vi "2B_Tech_TCP_Packet_TWBOZO_v1.1.vi"(7 "TCP Packet In":string, 12 "Data Array":string[](array[string])) -> (8 "TCP Binary Packet":string)   [LabVIEW 2014]
panel:
  out "array":string[](array[string])
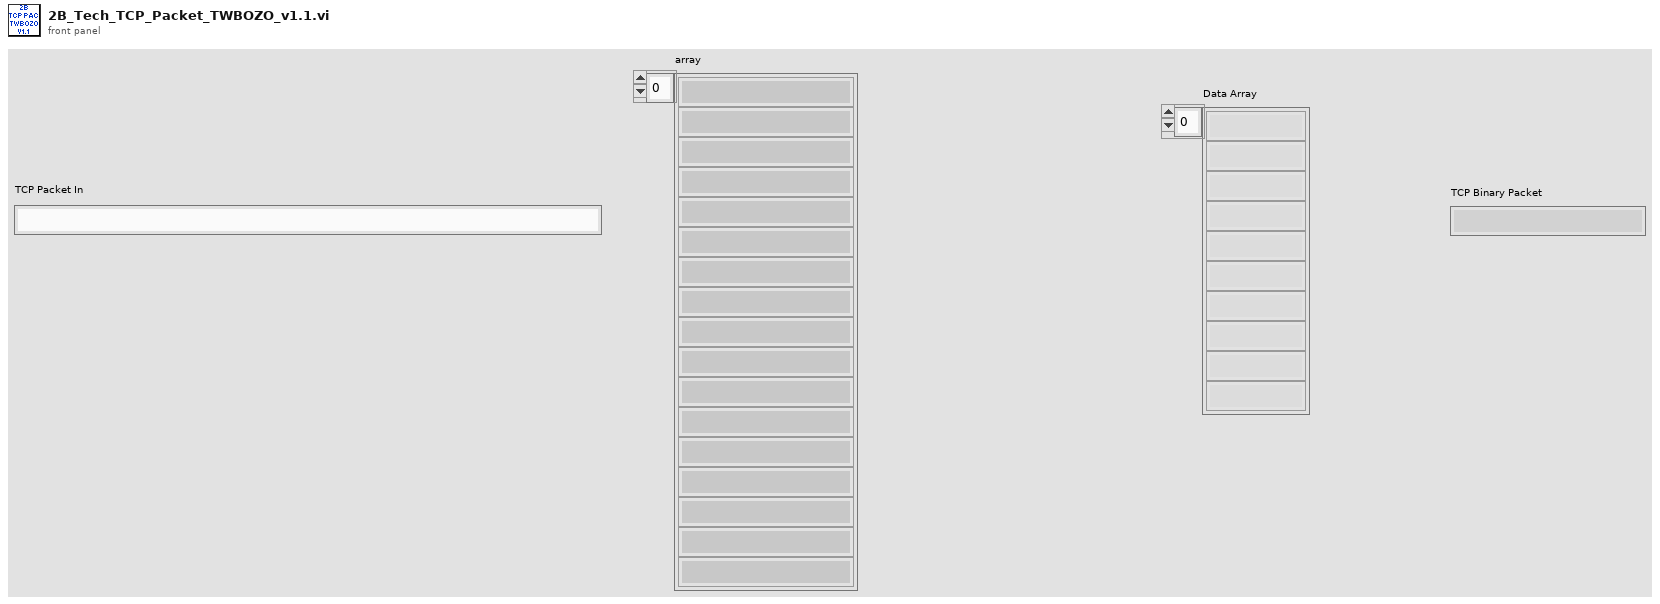
[diagram p1: front panel]
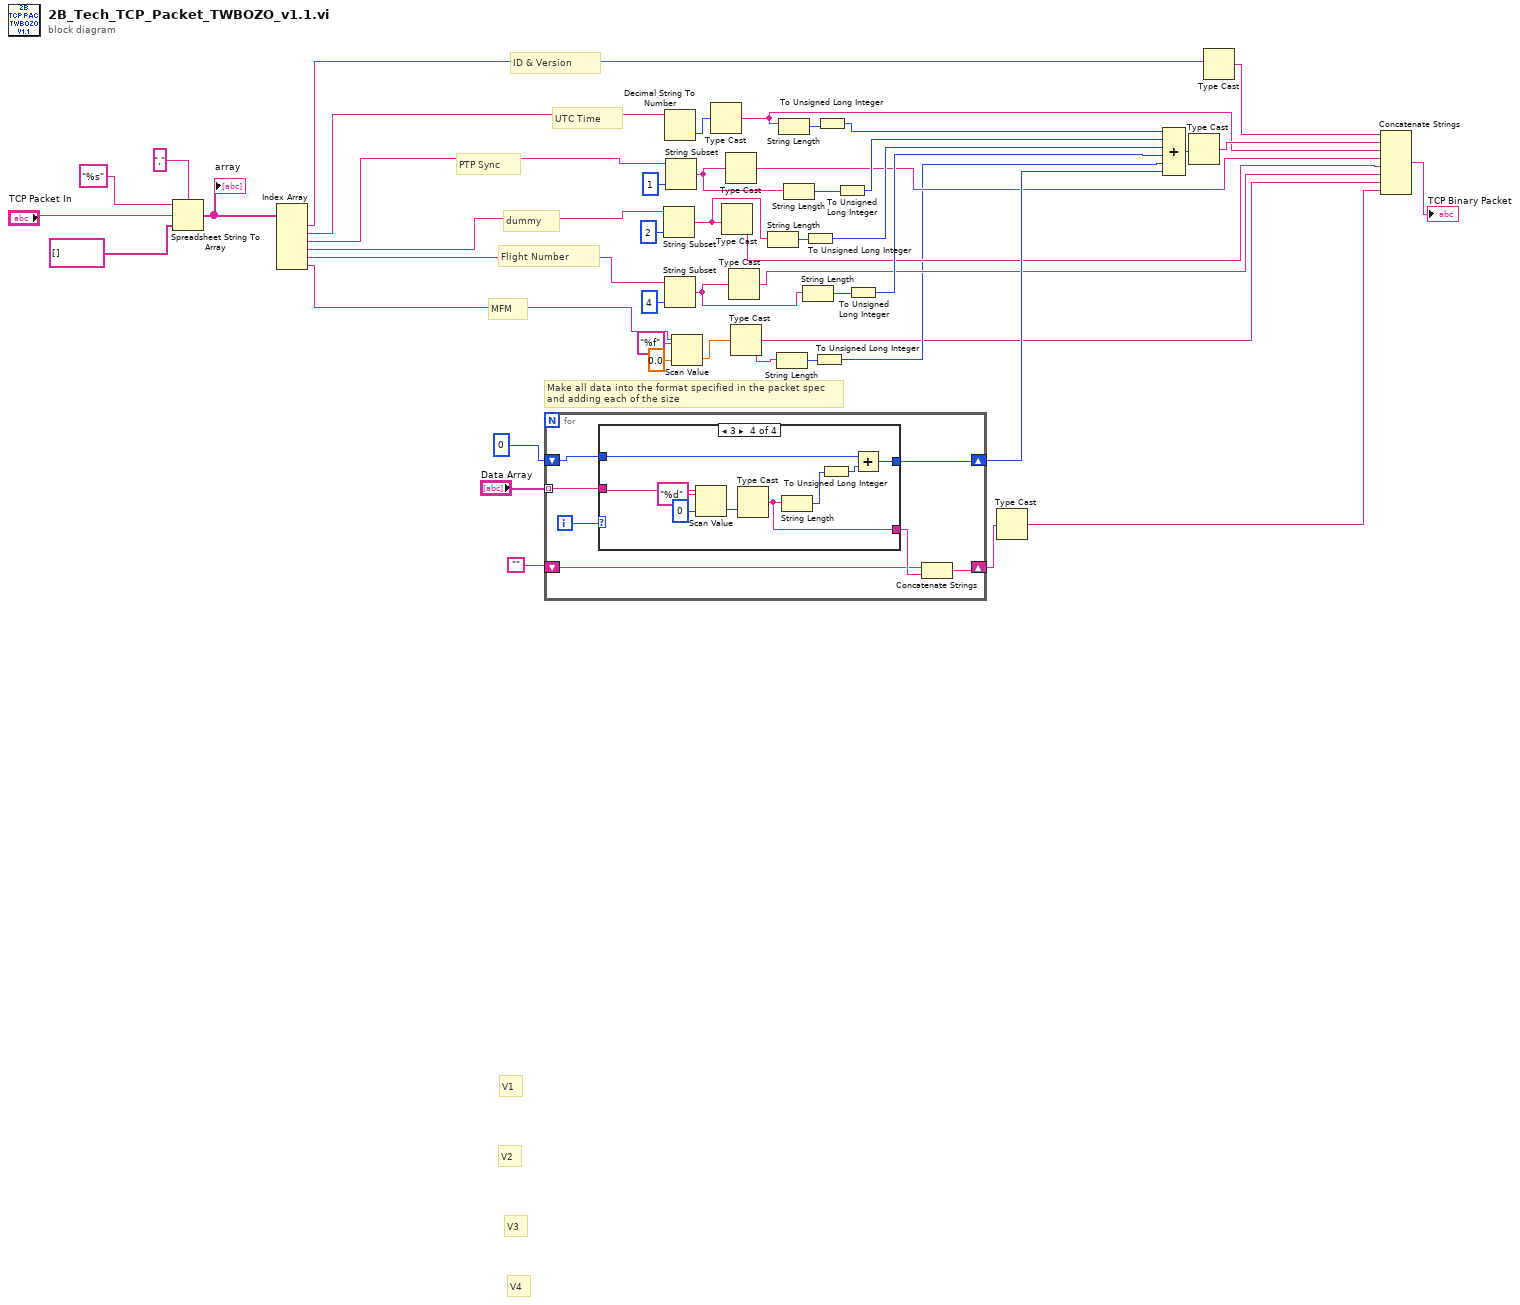
[diagram p0: block diagram]
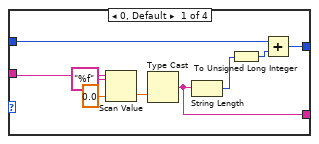
[diagram p2: hidden frame]
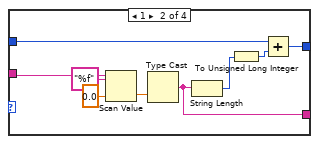
[diagram p3: hidden frame]
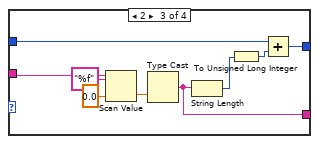
[diagram p4: hidden frame]
diagram:
  # "dummy"
  # "V4"
  # "V3"
  # "V2"
  # "V1"
  # "Flight Number"
  # "MFM"
  # "PTP Sync"
  # "UTC Time"
  # "ID & Version"
  # "Make all data into the format specified in the packet spec\nand adding each of the size"
  n1 = Spreadsheet String To Array(delimiter (Tab)=",", format string="%s", spreadsheet string="TCP Packet In", array type (2D Dbl)=string[] []) -> (array=w18:string[])
  "array" <- w18
  n2 = Index Array(array=w18) -> (element #1=w17:string, element #2=w2:string, element #3=w16:string, element #4=w5:string, element #5=w15:string, element #6=w9:string)  [unwired: 6 in]
  n3 = for {
    tunnel: "Data Array" -> [w52] mode=indexing
    shift-right: [w50] -> w34
    shift-left: u32 0 -> [w51]
    shift-right: [w49] -> w23
    shift-left: "" -> [w47]
    i -> [w53]
    n4 = case shown="3" w53 {
      tunnel: w52 -> [w60 w69 w78 w87]
      tunnel: w51 -> [w58 w67 w76 w85]
      tunnel: [w55 w64 w73 w82] -> w50
      tunnel: [w54 w63 w72 w81] -> w48
      frame 0, Default {
        n5 = Scan Value(string=w60, format string="%f", default (0 dbl)=sgl 0.0 ("default (0 I32)")) -> (value=w62:sgl)  [unwired: 1 out]
        n6 = Type Cast(x=w62) -> (*(type *) &x=w54:string)  [unwired: 1 in]
        n7 = String Length(string=w54) -> (length=w57:i32)
        n8 = To Unsigned Long Integer(number=w57) -> (unsigned 32bit integer=w56:u32)
        n9 = Add(x=w58, y=w56) -> (x+y=w55:u32)
      }
      frame 1 {
        n10 = Scan Value(string=w69, format string="%f", default (0 dbl)=sgl 0.0 ("default (0 I32)")) -> (value=w71:sgl)  [unwired: 1 out]
        n11 = Type Cast(x=w71) -> (*(type *) &x=w63:string)  [unwired: 1 in]
        n12 = String Length(string=w63) -> (length=w66:i32)
        n13 = To Unsigned Long Integer(number=w66) -> (unsigned 32bit integer=w65:u32)
        n14 = Add(x=w67, y=w65) -> (x+y=w64:u32)
      }
      frame 2 {
        n15 = Scan Value(string=w78, format string="%f", default (0 dbl)=sgl 0.0 ("default (0 I32)")) -> (value=w80:sgl)  [unwired: 1 out]
        n16 = Type Cast(x=w80) -> (*(type *) &x=w72:string)  [unwired: 1 in]
        n17 = String Length(string=w72) -> (length=w75:i32)
        n18 = To Unsigned Long Integer(number=w75) -> (unsigned 32bit integer=w74:u32)
        n19 = Add(x=w76, y=w74) -> (x+y=w73:u32)
      }
      frame 3 {
        n20 = Scan Value(string=w87, format string="%d", default (0 dbl)=0 ("default (0 I32)")) -> (value=w89:i32)  [unwired: 1 out]
        n21 = Type Cast(x=w89) -> (*(type *) &x=w81:string)  [unwired: 1 in]
        n22 = String Length(string=w81) -> (length=w84:i32)
        n23 = To Unsigned Long Integer(number=w84) -> (unsigned 32bit integer=w83:u32)
        n24 = Add(x=w85, y=w83) -> (x+y=w82:u32)
      }
    }
    n25 = Concatenate Strings(w47, w48) -> (w49:string)
  }
  n26 = String Subset(string=w5, length (rest)=2 ("length (rest)")) -> (substring=w4:string)  [unwired: 1 in]
  n27 = Decimal String To Number(string=w2) -> (number=w3:i32)  [unwired: 2 in, 1 out]
  n28 = String Subset(string=w15, length (rest)=4 ("length (rest)")) -> (substring=w27:string)  [unwired: 1 in]
  n29 = String Subset(string=w16, length (rest)=1 ("length (rest)")) -> (substring=w30:string)  [unwired: 1 in]
  n30 = Scan Value(string=w9, format string="%f", default (0 dbl)=sgl 0.0 ("default (0 I32)")) -> (value=w10:sgl)  [unwired: 1 out]
  n31 = Type Cast(x=w3) -> (*(type *) &x=w1:string)  [unwired: 1 in]
  n32 = Type Cast(x=w4) -> (*(type *) &x=w14:string)  [unwired: 1 in]
  n33 = Type Cast(x=w30) -> (*(type *) &x=w29:string)  [unwired: 1 in]
  n34 = Type Cast(x=w27) -> (*(type *) &x=w28:string)  [unwired: 1 in]
  n35 = Type Cast(x=w10) -> (*(type *) &x=w7:string)  [unwired: 1 in]
  n36 = String Length(string=w4) -> (length=w41:i32)
  n37 = String Length(string=w7) -> (length=w13:i32)
  n38 = String Length(string=w1) -> (length=w46:i32)
  n39 = String Length(string=w30) -> (length=w43:i32)
  n40 = String Length(string=w27) -> (length=w38:i32)
  n41 = To Unsigned Long Integer(number=w41) -> (unsigned 32bit integer=w40:u32)
  n42 = To Unsigned Long Integer(number=w13) -> (unsigned 32bit integer=w8:u32)
  n43 = To Unsigned Long Integer(number=w46) -> (unsigned 32bit integer=w45:u32)
  n44 = To Unsigned Long Integer(number=w43) -> (unsigned 32bit integer=w42:u32)
  n45 = To Unsigned Long Integer(number=w38) -> (unsigned 32bit integer=w37:u32)
  n46 = Type Cast(x=w23) -> (*(type *) &x=w26:string)  [unwired: 1 in]
  n47 = Compound Arithmetic op=ADD(w45, w42, w40, w37, w8, w34) -> (w32:u32)
  n48 = Type Cast(x=w32) -> (*(type *) &x=w31:string)  [unwired: 1 in]
  n49 = Type Cast(x=w17) -> (*(type *) &x=w33:string)  [unwired: 1 in]
  n50 = Concatenate Strings(w33, w31, w1, w29, w14, w28, w7, w26) -> (→"TCP Binary Packet":string)
